vi "CSM - Forward States to CSM.vi"(6 "High Priority? (T)":bool=TRUE, 7 "Module Name":string, 8 "Error In (No Error)":errorcluster, 11 "State (S) In (\"\")":string) -> (0 "error out":errorcluster)   [LabVIEW 2017, in "Communicable State Machine.lvlib"]
doc: "### CSM - Forward States to CSM.vi\n\n-- <b>Controls</b> --\n- <b>High Priority(T)</b>:\n- <b>Module Name</b>: Returns any argument(s) that may be used in the current state string. These arguments come after the \">>\" characters\n- <b>State(s) in (\"\")</b>: Wire the existing states to this input. The default is an empty string."
uses:
  Communicable State Machine.lvlib
  _Support/CSMQ/_CSMOFGVOPER.ctl
  _Support/Typedef/_Cross CSM State Data.ctl
  _Support/Typedef/_CSM_MSG_TYPE.ctl
  _Support/Typedef/_Cross CSM State Response.ctl
  _Support/Typedef/_CSM_Response Source Message.ctl
  _Shared/CSM Shared.lvlib
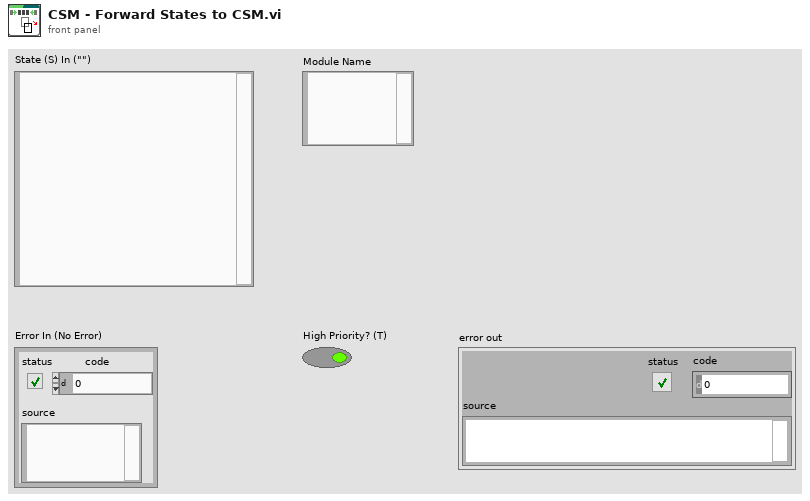
[diagram p1: front panel]
types:
  T1 = typedef "Communicable State Machine.lvlib/_CSM_MSG_TYPE.ctl" = enum16{"Sync Message(-@)", "Async Message(->)", "Async without Response(->|)", "Async Response", "Broadcast(-><all>)", "Broadcast(-><status>)", "Broadcast(-><interrupt>)", "Append to JKISM States", "Append to JKISM States(High Priority)", "Broadcast(-><state>)"}
  T2 = typedef "Communicable State Machine.lvlib/_Cross CSM State Data.ctl" = cluster{"Msg Type":T1, "state":string, "args":string, "source":string, "RespQ":refnum<queue>, "Response For Message":T3, "Target":string}
  T3 = typedef "Communicable State Machine.lvlib/_CSM_Response Source Message.ctl" = cluster{"‘State":string, "’Arguments":string, "’Error":errorcluster}
  T4 = typedef "Communicable State Machine.lvlib/_CSMOFGVOPER.ctl" = enum16{"Create If not Exist", "Get By Name", "List", "Check If Name Exists", "Release", "Module Status", "Create Status Event Handler", "Destroy Status Event Handler", "Clear Invalid Objs"}
  T5 = typedef "Communicable State Machine.lvlib/_CSMObj.ctl" = cluster{"info":T6, "Refs":T8}
  T6 = typedef "Communicable State Machine.lvlib/_CSMObj-Info.ctl" = cluster{"Module Name":string, "Requested Name":string, "Group Name":string, "Mode":T7, "Allowed Messages":string[]}
  T7 = typedef "Communicable State Machine.lvlib/_CSM_MODE.ctl" = enum16{"Not Exist", "Stand Alone", "CSM", "Worker", "Worker Agent", "Chain Node", "Chain"}
  T8 = typedef "Communicable State Machine.lvlib/_CSMObj-Refs.ctl" = cluster{"WatchDogQ":refnum<queue>, "CSMDataDVR":refnum<data-value>, "Queue":T9, "GroupDataDVR":refnum<data-value>, "TagMap":refnum<data-value>, "ExitEvent":refnum<user-event>, "NewStateEvent":refnum<user-event>, "StatusChangeEvent":refnum<user-event>}
  T9 = typedef "Communicable State Machine.lvlib/Priority Queue.ctl" = cluster{"HPriorityQ":refnum<queue>, "LowPriorityQ":refnum<queue>}
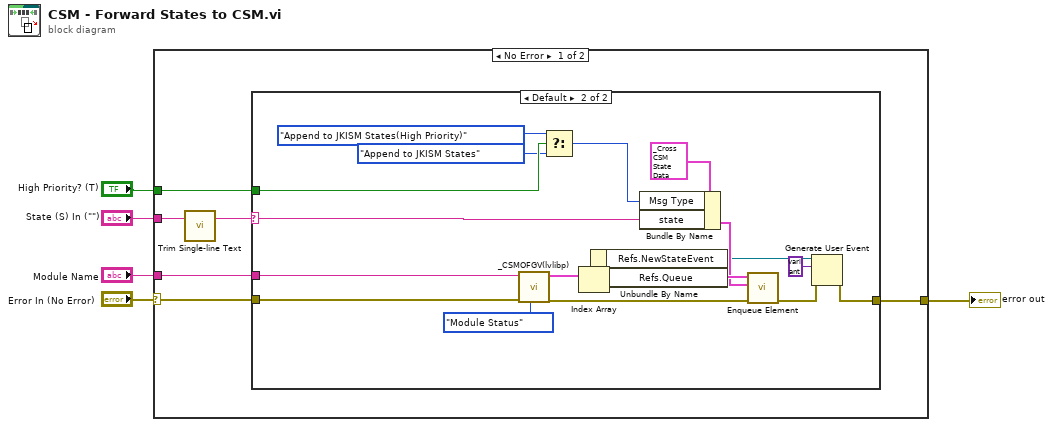
[diagram p0: block diagram]
diagram:
  n1 = case shown="No Error" "Error In (No Error)" {
    selector: "Error In (No Error)" -> [w10 w31]
    tunnel: "State (S) In (\"\")" -> [w9 _]
    tunnel: [w11 w31] -> w3
    tunnel: "Module Name" -> [w8 _]
    tunnel: "High Priority? (T)" -> [w7 _]
    frame No Error {
      n2 = call "Trim Single-line Text.vi"("single-line text"=w9) -> ("trimed text"=w6:string)  [unwired: 2 in]
      n3 = case shown="Default" w6 {
        selector: w6 -> [_ w27]
        tunnel: [w12 w13] -> w11
        tunnel: w10 -> [w12 w30]
        tunnel: w8 -> [_ w29]
        tunnel: w7 -> [_ w28]
        frame "" {
        }
        frame Default {
          n4 = call "_CSMOFGV(lvlibp).vi"("Operation"=_CSMOFGVOPER."Module Status", "Error In"=w30, "Name (\"\" to Use UUID) In"=w29) -> ("error out"=w20:errorcluster, "Array"=w25:T5[])  [unwired: 6 in, 1 out]
          n5 = Select(t=_CSM_MSG_TYPE."Append to JKISM States(High Priority)" ("Msg Type"), s=w28, f=_CSM_MSG_TYPE."Append to JKISM States" ("Msg Type")) -> (s? t:f=w19:T1)
          n6 = Index Array(array=w25) -> (element=w24:T5)  [unwired: 1 in]
          n7 = Unbundle By Name(w24) -> ("Refs.NewStateEvent"=w15:refnum<user-event>, "Refs.Queue"=w23:T9)
          n8 = Bundle By Name(cluster=T2 {"Msg Type"=enum."Sync Message(-@)", "state"="", "args"="", "source"="", "RespQ"=refnum, "Response For Message"={"‘State"="", "’Arguments"="", "’Error"={"status"=FALSE, "code"=0, "source"=""}}, "Target"=""} ("element"), "Msg Type"=w19, "state"=w27) -> (w21:T2)
          n9 = call "Enqueue Element.vi"("error in (no error)"=w20, "Cross JKI State Machine State"=w21, "Priority Queue"=w23) -> ("error out"=w14:errorcluster)  [unwired: 7 in, 1 out]
          n10 = Generate User Event(user event=w15, event data cluster=variant ("event data"), error in=w14) -> (error out=w13:errorcluster)  [unwired: 1 in, 1 out]
        }
      }
    }
    frame Error {
    }
  }
  "error out" <- w3
